vi "Configure Gate Stop.vi"(5 "Gate Stop Holdoff Time (0 s)":dbl, 6 "Gate Stop Holdoff Event (1)":dbl=1.0, 7 "Gate Stop Holdoff Source (1: Time)":i32(ring)=1 items=[" Immediate", "Time", "Events"], 8 "error in (no error)":errorcluster, 9 "Gate Stop Slop (1: Negative)":i32(ring)=1 items=["Positive", "Negative"], 10 "Gate Stop Source (0:  Immediate)":i32(ring) items=[" Immediate", " External"], 11 "VISA resource name":refnum<visa-resource-name>) -> (0 "error out":errorcluster, 3 "VISA resource name out":refnum<visa-resource-name>)   [LabVIEW 2024, in "Agilent 532XX Series.lvlib"]
doc: "Configures the advanced characteristics of gate stop.\n\n<B>Note:</B> This VI only applies to the Agilent 53220A/53230A."
uses:
  Agilent 532XX Series.lvlib
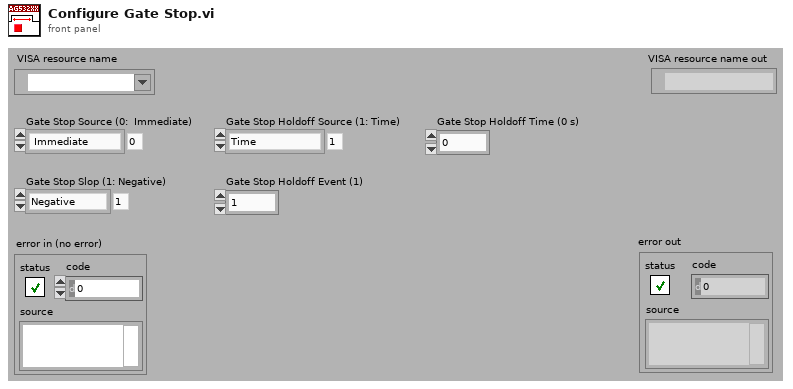
[diagram p1: front panel]
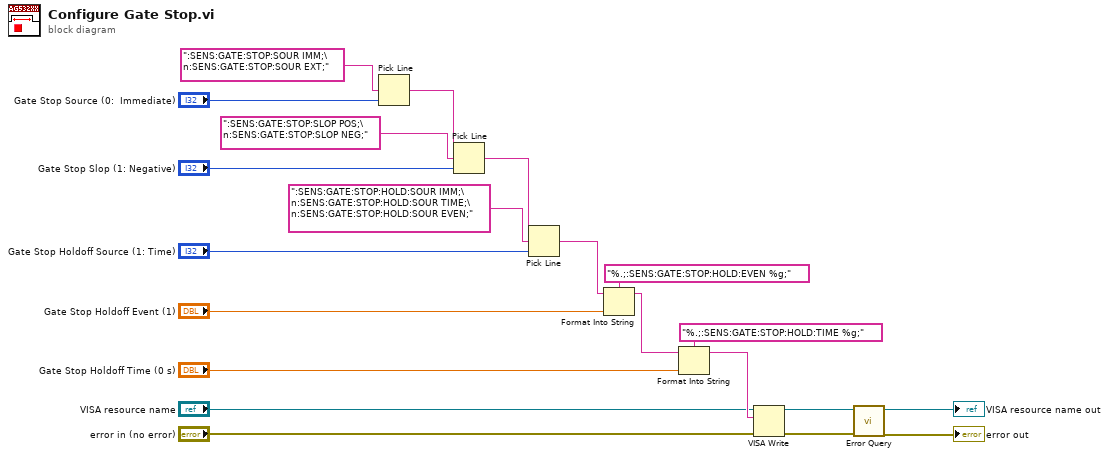
[diagram p0: block diagram]
diagram:
  n1 = Pick Line(multi-line string=":SENS:GATE:STOP:SOUR IMM;\n:SENS:GATE:STOP:SOUR EXT;", line index="Gate Stop Source (0:  Immediate)") -> (output string=w17:string)  [unwired: 1 out]
  n2 = Pick Line(string ("")=w17, multi-line string=":SENS:GATE:STOP:SLOP POS;\n:SENS:GATE:STOP:SLOP NEG;", line index="Gate Stop Slop (1: Negative)") -> (output string=w14:string)
  n3 = Pick Line(string ("")=w14, multi-line string=":SENS:GATE:STOP:HOLD:SOUR IMM;\n:SENS:GATE:STOP:HOLD:SOUR TIME;\n:SENS:GATE:STOP:HOLD:SOUR EVEN;", line index="Gate Stop Holdoff Source (1: Time)") -> (output string=w13:string)
  n4 = Format Into String(format string="%.;:SENS:GATE:STOP:HOLD:EVEN %g;", initial string=w13, "Gate Stop Holdoff Event (1)") -> (resulting string=w10:string)  [unwired: 1 in, 1 out]
  n5 = Format Into String(format string="%.;:SENS:GATE:STOP:HOLD:TIME %g;", initial string=w10, "Gate Stop Holdoff Time (0 s)") -> (resulting string=w7:string)  [unwired: 1 in, 1 out]
  n6 = VISA Write(VISA resource name="VISA resource name", write buffer=w7, error in (no error)="error in (no error)") -> (VISA resource name out=w4:refnum<visa-resource-name>, error out=w3:errorcluster)  [unwired: 1 out]
  n7 = call "Error Query.vi"("error in (no error)"=w3, "VISA resource name"=w4) -> ("error out"=→"error out":errorcluster, "VISA resource name out"=→"VISA resource name out":refnum<visa-resource-name>)  [unwired: 8 out]
